vi "Parse Response-JSONtext.vi"(8 "error in (no error)":errorcluster, 10 "{JSON} Response":string) -> (0 "error out":errorcluster, 2 "result":string, 4 "id":string)   [LabVIEW 2019, in "JSON-RPC.lvclass"]
uses:
  JSON-RPC.lvclass
  typedefs/Error--Cluster.ctl
  7ce7fba8-9f44-478d-b6cb-b571ff29f2f5.vi
  8c905beb-ab4c-49e3-b5c6-2c663b7b30d7.vi
  fce5892e-0c40-47e1-88e0-6c122aadefe2.vi
  <vilib>/JDP Science/JSONtext/Find Item.vi
  <vilib>/JDP Science/JSONtext/Next JSON Value.vi
  <vilib>/JDP Science/JSONtext/String Subset.vi
  <vilib>/JDP Science/JSONtext/Parsing/Advance past next JSON Value (inlined COPY).vi
  <vilib>/JDP Science/JSONtext/Parsing/Advance past whitespace.vi
  <vilib>/JDP Science/JSONtext/Parsing/Advance past String.vi
  <vilib>/JDP Science/JSONtext/Parsing/Advance past Number.vi
  <vilib>/JDP Science/JSONtext/Parsing/Advance past Line Ending.vi
  <vilib>/JDP Science/JSONtext/Parsing/Parse Full Path or Item Name.vi
  <vilib>/JDP Science/JSONtext/Parsing/Advance past Array.vi
  <vilib>/JDP Science/JSONtext/Parsing/Advance past Object.vi
  <vilib>/JDP Science/JSONtext/support/Error Cluster From Code.vi
  <vilib>/JDP Science/JSONtext/Offset/Find Item Locations by Path.vi
  <vilib>/JDP Science/JSONtext/JSON text to Variant.vi
  <vilib>/JDP Science/JSONtext/LVClass Serializer/JSONtext LVClass Serializer.lvclass
  <vilib>/JDP Science/JSONtext/JSONtext.lvlib
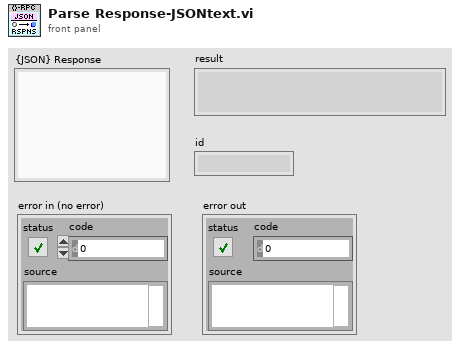
[diagram p1: front panel]
types:
  T1 = cluster{"jsconrpc":string, "result":string, "id":string}
  T2 = typedef "JSON-RPC.lvclass/Error--Cluster.ctl" = cluster{"code":i32, "message":string}
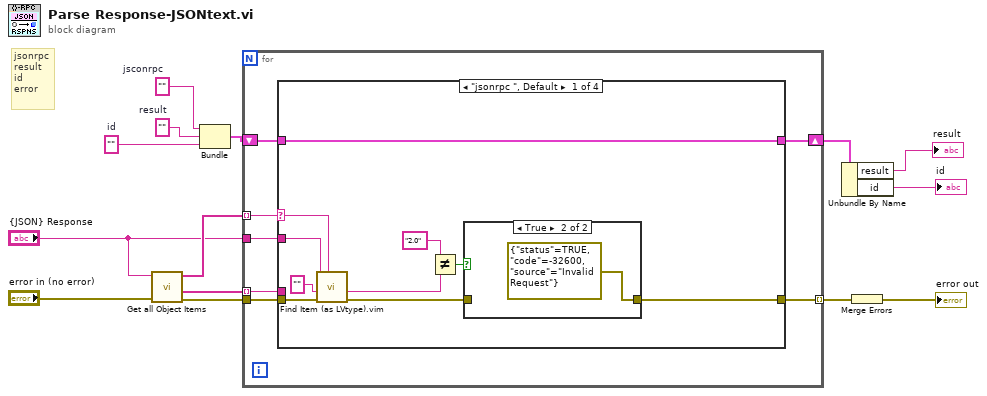
[diagram p0: block diagram]
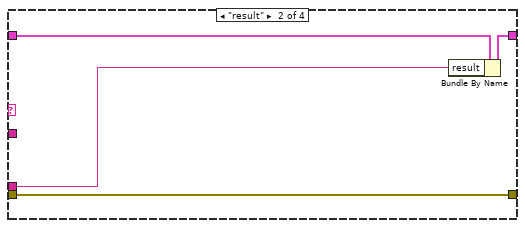
[diagram p3: hidden frame]
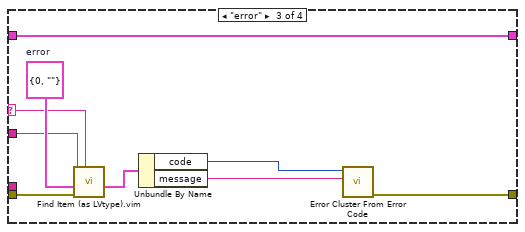
[diagram p4: hidden frame]
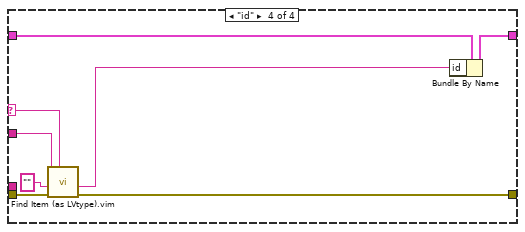
[diagram p5: hidden frame]
diagram:
  w12 = ""  # id
  w11 = ""  # jsconrpc
  w10 = ""  # result
  # "jsonrpc\nresult\nid\nerror"
  n1 = call <vilib>:"Get all Object Items.vi"("error in (no error)"="error in (no error)", "JSON"="{JSON} Response") -> ("error out"=w7:errorcluster, "<JSON>"=w6:string[], "Item Names"=w9:string[])  [unwired: 6 in, 1 out]
  n2 = Bundle("jsconrpc"=w11, "result"=w10, "id"=w12) -> (w13:T1)  [unwired: 1 in]
  n3 = for {
    tunnel: w6 -> [w20] mode=indexing
    tunnel: w9 -> [w21] mode=indexing
    tunnel: w7 -> [w19]
    tunnel: [w18] -> w8 mode=indexing
    tunnel: "{JSON} Response" -> [w17]
    shift-right: [w15] -> w14
    shift-left: w13 -> [w16]
    n4 = case shown="\"jsonrpc \", Default" w21 {
      selector: w21 -> [w26 _ w42 w54]
      tunnel: w20 -> [_ w35 _ _]
      tunnel: w19 -> [w28 w34 w44 w53]
      tunnel: [w29 w34 w38 w52] -> w18
      tunnel: w17 -> [w22 _ w43 w47]
      tunnel: w16 -> [w23 w37 w46 w50]
      tunnel: [w23 w36 w46 w49] -> w15
      frame "jsonrpc ", Default {
        n5 = call "Find Item (as LVtype).vim"("$Path or Item Name"=w26, "error in (no error)"=w28, "Data Type and Default Value"="" ("x"), "JSON"=w22) -> ("error out"=w27:errorcluster, "Data"=w25:string)  [unwired: 4 in, 2 out]
        n6 = Not Equal?(x="2.0", y=w25) -> (x != y?=w30:bool)
        n7 = case shown="True" w30 {
          tunnel: w27 -> [w32 _]
          tunnel: [w32 errorcluster {"status"=TRUE, "code"=-32600, "source"="Invalid Request"} ("error out")] -> w29
          frame False {
          }
          frame True {
          }
        }
      }
      frame "result" {
        n8 = Bundle By Name(cluster=w37, "result"=w35) -> (w36:T1)
      }
      frame "error" {
        w45 = T2 {"code"=0, "message"=""}  # error
        n9 = call "Find Item (as LVtype).vim"("$Path or Item Name"=w42, "error in (no error)"=w44, "Data Type and Default Value"=w45, "JSON"=w43) -> ("Data"=w41:T2)  [unwired: 4 in, 3 out]
        n10 = Unbundle By Name(w41) -> ("code"=w40:i32, "message"=w39:string)
        n11 = call <vilib>:"Error Cluster From Error Code.vi"("error message (\"\")"=w39, "error code (0)"=w40) -> ("error out"=w38:errorcluster)  [unwired: 7 in]
      }
      frame "id" {
        n12 = call "Find Item (as LVtype).vim"("$Path or Item Name"=w54, "error in (no error)"=w53, "Data Type and Default Value"="", "JSON"=w47) -> ("error out"=w52:errorcluster, "Data"=w48:string)  [unwired: 4 in, 2 out]
        n13 = Bundle By Name(cluster=w50, "id"=w48) -> (w49:T1)
      }
    }
  }
  n14 = Unbundle By Name(w14) -> ("result"=→"result":string, "id"=→"id":string)
  n15 = Merge Errors(w8) -> (→"error out":errorcluster)
